vi "N07_State_Machine.vi"() -> ()   [LabVIEW 2023]
panel:
  out "String":string
  in  "Next State":bool
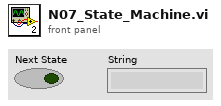
[diagram p1: front panel]
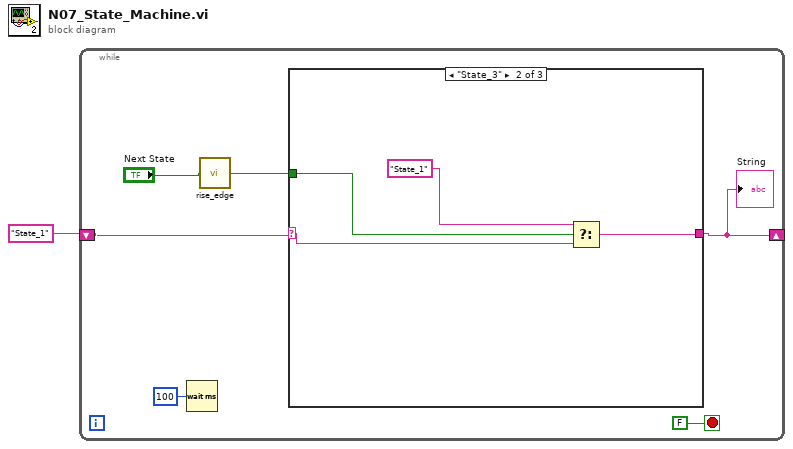
[diagram p0: block diagram]
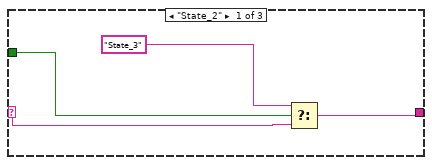
[diagram p2: hidden frame]
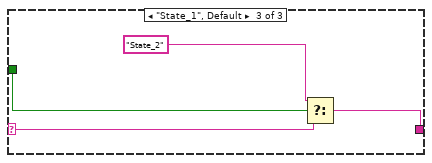
[diagram p3: hidden frame]
diagram:
  n1 = while {
    shift-right: [w3] -> _
    shift-left: "State_1" -> [w7]
    stop <- FALSE stop-if-true
    n2 = Wait (ms)(milliseconds to wait=u32 100) -> ()  [unwired: 1 out]
    n3 = call "rise_edge.vi"("In"="Next State") -> ("Out"=w4:bool)
    n4 = case shown="\"State_3\"" w7 {
      selector: w7 -> [w11 w13 w19]
      tunnel: [w10 w12 w16] -> w3
      tunnel: w4 -> [w8 w14 w18]
      frame "State_2" {
        n5 = Select(t="State_3", s=w8, f=w11) -> (s? t:f=w10:string)
      }
      frame "State_3" {
        n6 = Select(t="State_1", s=w14, f=w13) -> (s? t:f=w12:string)
      }
      frame "State_1", Default {
        n7 = Select(t="State_2", s=w18, f=w19) -> (s? t:f=w16:string)
      }
    }
    "String" <- w3
  }
